vi "SHIFT SETTING.vi"() -> ()   [LabVIEW 2017]
uses:
  <vilib>/addons/database/Connection.llb/DB Tools Open Connec (String).vi
  <vilib>/addons/database/Auxilliary.llb/DB Tools Format Datetime String (Time Stamp).vi
  <vilib>/addons/database/NI_Database_API.lvlib
panel:
  in  "error in (no error)":errorcluster
  out "error out":errorcluster
  in  "Save":bool
  in  "1Start":timestamp format="%<%H:%M:%S>T"
  in  "2Start":timestamp format="%<%H:%M:%S>T"
  in  "3Start":timestamp format="%<%H:%M:%S>T"
  in  "2End":timestamp format="%<%H:%M:%S>T"
  in  "3End":timestamp format="%<%H:%M:%S>T"
  in  "1End":timestamp format="%<%H:%M:%S>T"
  in  "Exit":bool
  # "Start Time"
  # "End Time"
  # "Shift 1"
  # "Shift 2"
  # "Shift 3"
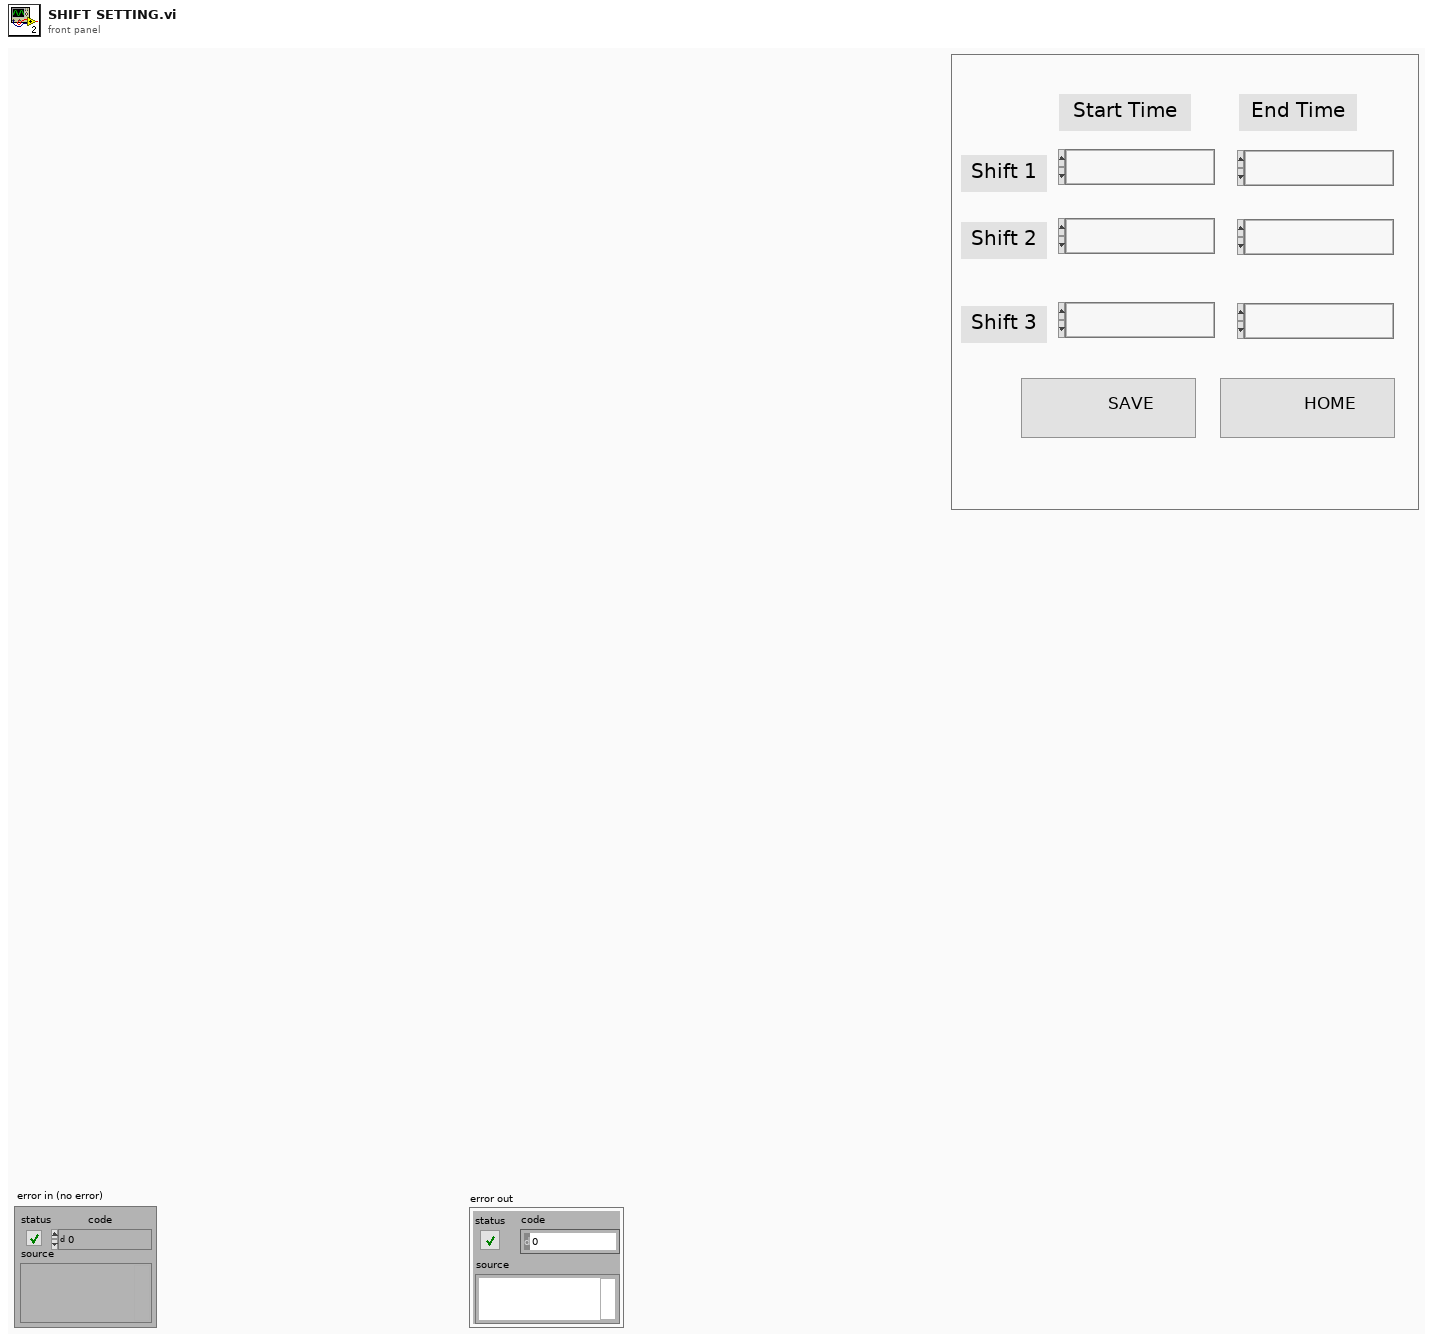
[diagram p1: front panel]
types:
  T1 = typedef "NI_Database_API.lvlib/Conn ObjectReference.ctl" = refnum<k1>
  T2 = enum32{"invalid app kind", "Development System", "Run Time System", "Student Edition", "Embedded LabVIEW", "Evaluation", "Custom"}
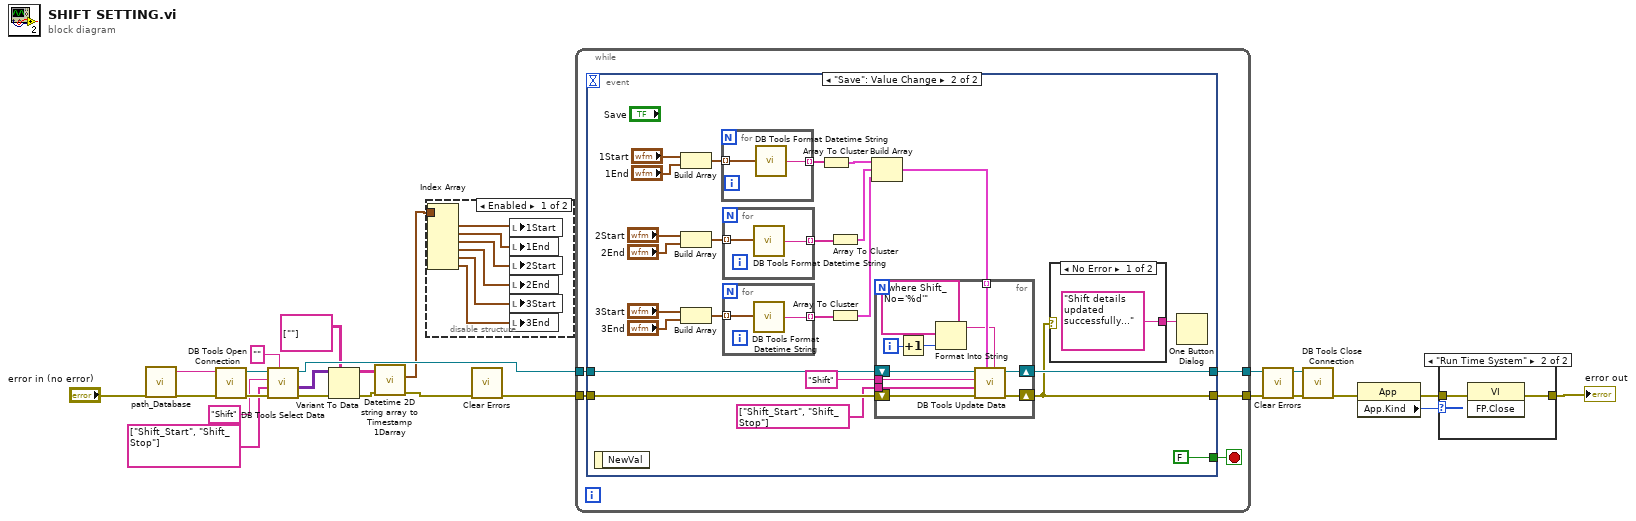
[diagram p0: block diagram]
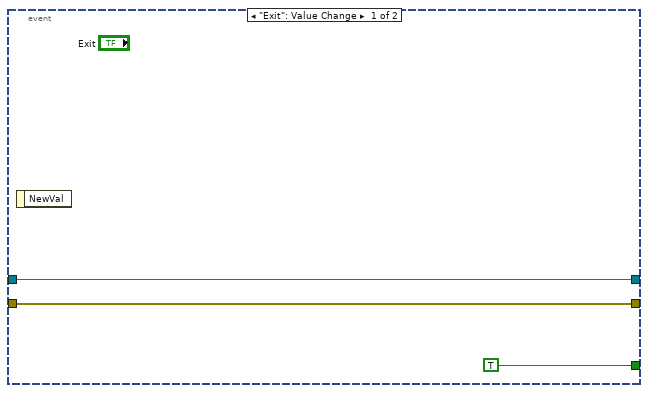
[diagram p4: hidden frame]
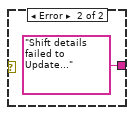
[diagram p5: hidden frame]
diagram:
  n1 = call "path_Database.vi"("error in"="error in (no error)") -> ("error out"=w10:errorcluster, "resulting string"=w9:string)  [unwired: 9 in]
  n2 = call-poly <vilib>:"DB Tools Open Connection.vi"("error in (no error)"=w10, "connection information"=w9) -> ("error out"=w23:errorcluster, "connection reference"=w24:T1)  [unwired: 6 in]
  n3 = call <vilib>:"DB Tools Select Data.vi"("condition"="", "error in (no error)"=w23, "columns"=string[] ["Shift_Start", "Shift_Stop"], "table"="Shift", "connection reference"=w24) -> ("error out"=w14:errorcluster, "data"=w16:variant[][], "connection reference out"=w19:T1)  [unwired: 1 in]
  n4 = Variant To Data(error in=w14, type=string[][] [[""]], Variant=w16) -> (data=w6:string[][], error out=w8:errorcluster)
  n5 = call "Datetime 2D string array to Timestamp 1Darray.vi"("error in (no error)"=w8, "String Array In"=w6) -> ("error out"=w7:errorcluster, "Time Stamp Out"=w5:timestamp[])  [unwired: 8 in]
  n6 = disable-structure shown="Enabled" {
    disable-tunnel: w5 -> [w31 _]
    frame Enabled {
      n7 = Index Array(array=w31) -> (element #1=w30:timestamp, element #2=w29:timestamp, element #3=w28:timestamp, element #4=w27:timestamp, element #5=w26:timestamp, element #6=w25:timestamp)  [unwired: 6 in]
      n8 = local write "1Start"(w30) -> ()
      n9 = local write "1End"(w29) -> ()
      n10 = local write "2Start"(w28) -> ()
      n11 = local write "2End"(w27) -> ()
      n12 = local write "3Start"(w26) -> ()
      n13 = local write "3End"(w25) -> ()
    }
    frame Disabled {
    }
  }
  n14 = call <vilib>:"Clear Errors.vi"("error in (no error)"=w7) -> ("error out"=w13:errorcluster)  [unwired: 5 in, 1 out]
  n15 = while {
    tunnel: w13 -> [w36]
    tunnel: [w35] -> w17
    tunnel: w19 -> [w33]
    tunnel: [w32] -> w18
    stop <- w34 stop-if-true
    n16 = event shown="[1] \"Save\": Value Change" {
      selector: _ -> [_ _]
      dyn-events: _ -> [_ _]
      timeout: _ -> [_ _]
      tunnel: w36 -> [w39 w62]
      tunnel: [w39 w41] -> w35
      tunnel: [TRUE FALSE] -> w34
      tunnel: w33 -> [w37 w63]
      tunnel: [w37 w61] -> w32
      event "Exit": Value Change {
        n17 = event-data() -> ()  [unwired: 1 in, 1 out]
      }
      event "Save": Value Change {
        n18 = event-data() -> ()  [unwired: 1 in, 1 out]
        n19 = Build Array("1Start", "1End") -> (w58:timestamp[])
        n20 = Build Array("2Start", "2End") -> (w53:timestamp[])
        n21 = Build Array("3Start", "3End") -> (w52:timestamp[])
        n22 = for {
          tunnel: w58 -> [w82] mode=indexing
          tunnel: [w81] -> w57 mode=indexing
          n23 = call-poly <vilib>:"DB Tools Format Datetime String.vi"("time stamp"=w82) -> ("date/time string"=w81:string)
        }
        n24 = for {
          tunnel: w53 -> [w80] mode=indexing
          tunnel: [w79] -> w54 mode=indexing
          n25 = call-poly <vilib>:"DB Tools Format Datetime String.vi"("time stamp"=w80) -> ("date/time string"=w79:string)
        }
        n26 = for {
          tunnel: w52 -> [w78] mode=indexing
          tunnel: [w77] -> w51 mode=indexing
          n27 = call-poly <vilib>:"DB Tools Format Datetime String.vi"("time stamp"=w78) -> ("date/time string"=w77:string)
        }
        n28 = Array To Cluster(array=w57) -> (cluster=w46:cluster{"[0]":string, "[1]":string})
        n29 = Array To Cluster(array=w54) -> (cluster=w45:cluster{"[0]":string, "[1]":string})
        n30 = Array To Cluster(array=w51) -> (cluster=w44:cluster{"[0]":string, "[1]":string})
        n31 = Build Array(w46, w45, w44) -> (w43:cluster{"[0]":string, "[1]":string}[])
        n32 = for {
          tunnel: "Shift" ("table") -> [w73]
          tunnel: string[] ["Shift_Start", "Shift_Stop"] ("columns") -> [w72]
          shift-right: [w67] -> w61
          shift-left: w63 -> [w76]
          shift-right: [w74] -> w41
          shift-left: w62 -> [w75]
          tunnel: w43 -> [w71] mode=indexing
          i -> [w70]
          n33 = Increment(x=w70) -> (x+1=w68:i32)
          n34 = Format Into String(format string="where Shift_No='%d'", w68) -> (resulting string=w66:string)  [unwired: 2 in, 1 out]
          n35 = call <vilib>:"DB Tools Update Data.vi"("condition"=w66, "data"=w71, "error in (no error)"=w75, "columns"=w72, "table"=w73, "connection reference"=w76) -> ("error out"=w74:errorcluster, "connection reference out"=w67:T1)  [unwired: 4 in]
        }
        n36 = case shown="No Error" w41 {
          tunnel: ["Shift details updated successfully..." "Shift details failed to Update..."] -> w40
          frame No Error {
          }
          frame Error {
          }
        }
        n37 = One Button Dialog(message=w40) -> ()  [unwired: 1 in, 1 out]
      }
    }
  }
  n38 = call <vilib>:"Clear Errors.vi"("error in (no error)"=w17) -> ("error out"=w12:errorcluster)  [unwired: 5 in, 1 out]
  n39 = call <vilib>:"DB Tools Close Connection.vi"("error in (no error)"=w12, "connection reference"=w18) -> ("error out"=w2:errorcluster)  [unwired: 5 in]
  n40 = property class="App"(error in=w2) -> (error out=w3:errorcluster, "App.Kind"=w4:T2)  [unwired: 1 in, 1 out]
  n41 = case shown="\"Run Time System\"" w4 {
    tunnel: w3 -> [w83 w85]
    tunnel: [w83 w84] -> w1
    frame Default {
    }
    frame "Run Time System" {
      n42 = invoke class="VI" method="FP.Close"(error in=w85) -> (error out=w84:errorcluster)  [unwired: 2 in, 2 out]
    }
  }
  "error out" <- w1
